vi "oax_Sound Reset.vi"(6 "Sound to Play":u16(ring) items=["Original", "Extracted", "Residue"], 8 "error in (no error)":errorcluster, 9 "Order waveform":waveform(dbl)[](array[waveform]), 10 "Vibration signals":waveform(dbl)[](array[waveform]), 11 "Order waveform":refnum<vi>) -> (0 "error out":errorcluster, 2 "Order Waveform Out":waveform(dbl)[](array[waveform]), 3 "task ID out":T1 format="%.0x")   [LabVIEW 2017]
uses:
  <vilib>/sound2/lvsound2.llb/Sound Output Task ID.ctl
  <vilib>/sound2/lvsound2.llb/Sampling Mode.ctl
  <vilib>/sound2/lvsound2.llb/Sound Output Write (DBL Single).vi
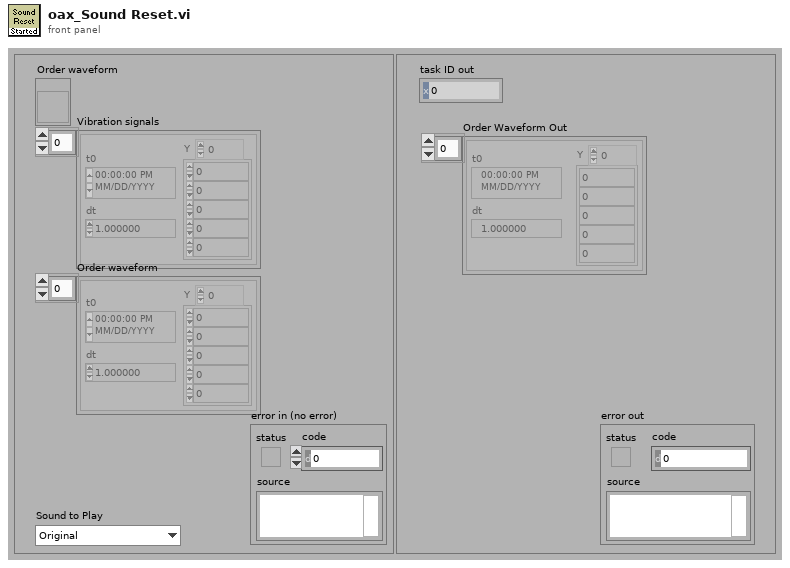
[diagram p1: front panel]
types:
  T1 = typedef "Sound Output Task ID.ctl" = u32
  T2 = typedef "Sampling Mode.ctl" = i32
  T3 = cluster{"Fs":dbl, "number of channels":i32, "bits per sample":i32}
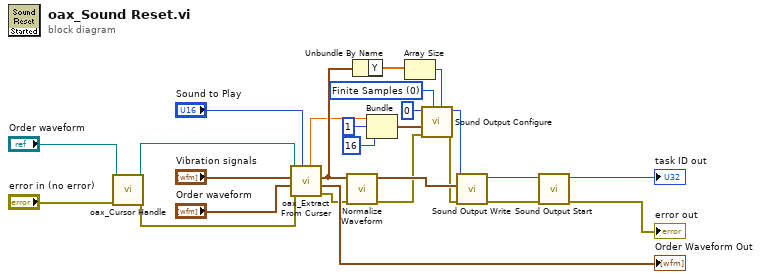
[diagram p0: block diagram]
diagram:
  w3 = T2 0 items=["Finite Samples", "Continuous Samples"] ("sample mode")
  n1 = call <vilib>:"oax_Cursor Handle.vi"("error in (no error)"="error in (no error)", "Order waveform"="Order waveform") -> ("error out"=w6:errorcluster, "Order waveform out"=w7:refnum<vi>)  [unwired: 8 in]
  n2 = call <vilib>:"oax_Extract From Curser.vi"("Sound to Play"="Sound to Play", "error in (no error)"=w6, 9:"Order waveform"="Order waveform", "Vibration signals"="Vibration signals", 11:"Order waveform"=w7) -> ("error out"=w12:errorcluster, "Order Waveform Out"=→"Order Waveform Out":waveform(dbl)[], "waveform out"=w5:waveform(dbl), "Fs"=w2:dbl)  [unwired: 2 in, 1 out]
  n3 = call <vilib>:"Normalize Waveform.vi"("error in (no error)"=w12, "waveform in"=w5) -> ("error out"=w11:errorcluster, "normalized waveform"=w13:waveform(dbl))  [unwired: 6 in, 2 out]
  n4 = Unbundle By Name(w5) -> ("Y"=w4:dbl[])
  n5 = Bundle("Fs"=w2, "number of channels"=1, "bits per sample"=16) -> (w15:T3)  [unwired: 1 in]
  n6 = Array Size(array=w4) -> (size(s)=w1:i32)
  n7 = call <vilib>:"Sound Output Configure.vi"("number of samples/ch"=w1, "sample mode"=w3, "error in (no error)"=w11, "sound format"=w15, "device ID"=u32 0) -> ("error out"=w10:errorcluster, "task ID"=w14:T1)  [unwired: 5 in]
  n8 = call-poly <vilib>:"Sound Output Write.vi"("error in (no error)"=w10, "data"=w13, "task ID"=w14) -> ("error out"=w20:errorcluster, "task ID out"=w19:T1)  [unwired: 7 in]
  n9 = call <vilib>:"Sound Output Start.vi"("error in (no error)"=w20, "task ID"=w19) -> ("error out"=→"error out":errorcluster, "task ID out"=→"task ID out":T1)  [unwired: 8 in]
